vi "Scale Channels.vi"(7 "Config":T1[](array[typedef]), 8 "error in (no error)":errorcluster, 11 "Channels In":dbl[](array[numeric])) -> (0 "error out":errorcluster, 3 "Channels Out":dbl[](array[numeric]))   [LabVIEW 2015]
doc: "This VI scales all raw channel outputs with gain and offset. Gain is multiplicative while offset is additive"
uses:
  Controls/Channel Configuration.ctl
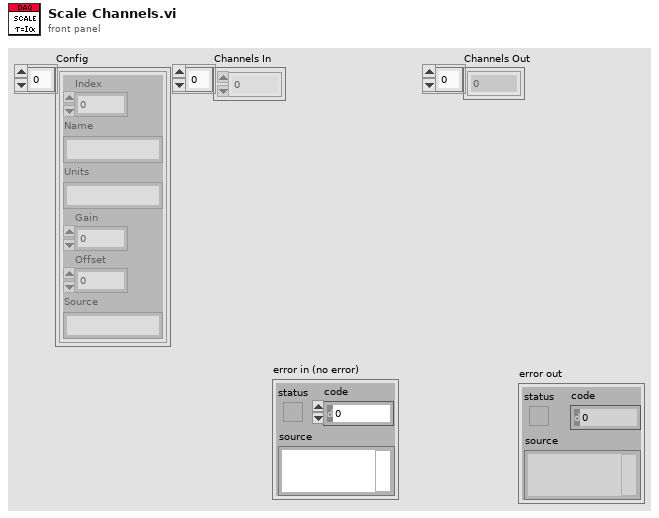
[diagram p1: front panel]
types:
  T1 = typedef "Channel Configuration.ctl" = cluster{"Index":u16, "Name":string, "Units":string, "Gain":dbl, "Offset":dbl, "Source":string}
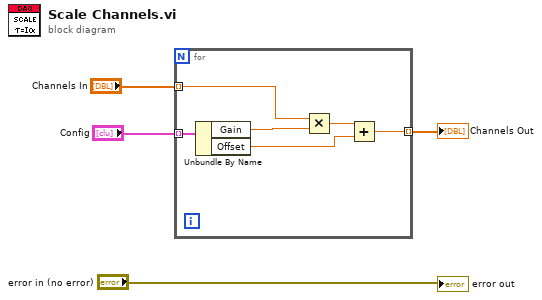
[diagram p0: block diagram]
diagram:
  n1 = for {
    tunnel: "Config" -> [w10] mode=indexing
    tunnel: "Channels In" -> [w9] mode=indexing
    tunnel: [w5] -> w1 mode=indexing
    n2 = Unbundle By Name(w10) -> ("Gain"=w8:dbl, "Offset"=w6:dbl)
    n3 = Multiply(x=w9, y=w8) -> (x*y=w7:dbl)
    n4 = Add(x=w7, y=w6) -> (x+y=w5:dbl)
  }
  "Channels Out" <- w1
  "error out" <- "error in (no error)"
